vi "Read Self Actor.vi"(11 "Process in":refnum<class "Process.lvclass">) -> (2 "Self Actor":refnum<class "LVCAM.lvclass">)   [LabVIEW 2021, in "Process.lvlib" / "Process.lvclass"]
uses:
  Process.lvclass
  LVCAM/LVCAM/LVCAM/LVCAM.lvclass
  Process.lvclass/Process.ctl
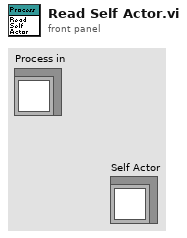
[diagram p1: front panel]
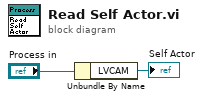
[diagram p0: block diagram]
diagram:
  n1 = Unbundle By Name("Process in") -> ("LVCAM"=→"Self Actor":refnum<class "LVCAM.lvclass">)
